vi "Initialize Transfers.vi"(7 "enable buffer conversion":bool, 8 "error in (no error)":errorcluster, 11 "transfer configurations":T1[](array[typedef]) {"channels"."string offset" format="%d bytes"}) -> (0 "error out":errorcluster, 3 "transfers":T6[](array[typedef]))   [LabVIEW 2017, in "DSF Core.lvlib" / "DSF PXImc Transceiver.lvclass"]
uses:
  DSF PXImc Transceiver.lvclass
  PXImc Transfer Data.ctl
  Typedefs/DSF Engine Transfer Configuration.ctl
  Typedefs/DSF Byte Order.ctl
  Typedefs/DSF Settings Info.ctl
  Typedefs/DSF Engine Channel Configuration.ctl
  Typedefs/DSF Data Type.ctl
  Classes/Configuration/Required Buffer Size (Transfer).vi
  Bad Setting Error.vi
  Classes/Configuration/Configuration Session.lvclass
  DSF Core.lvlib
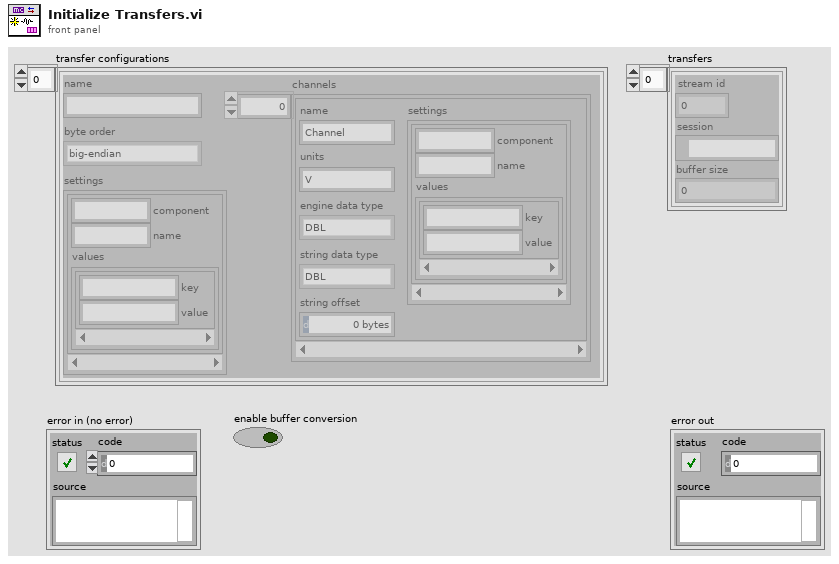
[diagram p1: front panel]
types:
  T1 = typedef "DSF Core.lvlib/DSF Engine Transfer Configuration.ctl" = cluster{"name":string, "byte order":T2, "settings":T3, "channels":T4[]}
  T2 = typedef "DSF Core.lvlib/DSF Byte Order.ctl" = enum8{"big-endian", "little-endian"}
  T3 = typedef "DSF Core.lvlib/DSF Settings Info.ctl" = cluster{"component":string, "name":string, "values":cluster{"key":string, "value":string}[]}[]
  T4 = typedef "DSF Core.lvlib/DSF Engine Channel Configuration.ctl" = cluster{"string offset":u64, "name":string, "units":string, "engine data type":T5, "string data type":T5, "settings":T3}
  T5 = typedef "DSF Core.lvlib/DSF Data Type.ctl" = enum8{"Bool", "SGL", "DBL", "I8", "I16", "I32", "I64", "U8", "U16", "U32", "U64"}
  T6 = typedef "DSF Core.lvlib/DSF PXImc Transceiver.lvclass/PXImc Transfer Data.ctl" = cluster{"stream id":u16, "session":refnum<k21>, "buffer size":u64}
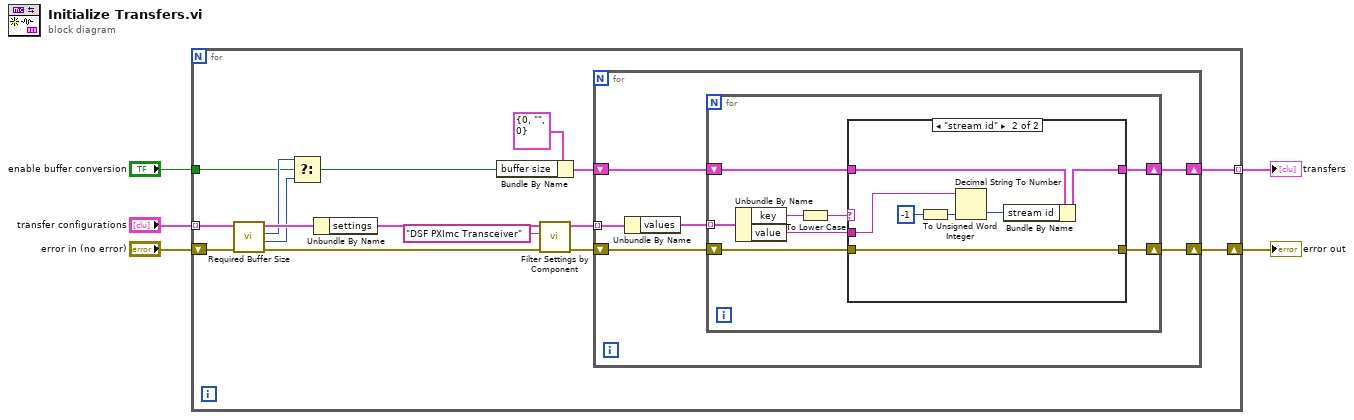
[diagram p0: block diagram]
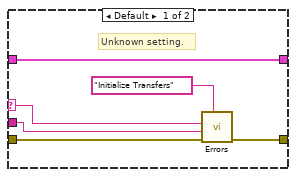
[diagram p2: hidden frame]
diagram:
  n1 = for {
    tunnel: "transfer configurations" -> [w13] mode=indexing
    tunnel: [w17] -> w3 mode=indexing
    shift-right: [w16] -> w4
    shift-left: "error in (no error)" -> [w12]
    tunnel: "enable buffer conversion" -> [w7]
    n2 = call-poly "Required Buffer Size.vi"("error in (no error)"=w12, "Transfer Configuration in"=w13) -> ("error out"=w10:errorcluster, "engine buffer size"=w8:u64, "string buffer size"=w9:u64, "Transfer Configuration out"=w11:T1)  [unwired: 6 in]
    n3 = Select(t=w9, s=w7, f=w8) -> (s? t:f=w6:u64)
    n4 = Unbundle By Name(w11) -> ("settings"=w21:T3)
    n5 = Bundle By Name(cluster=T6 {"stream id"=0, "session"="", "buffer size"=0} ("PXImc Transfer"), "buffer size"=w6) -> (w14:T6)
    n6 = call "Filter Settings by Component.vi"("error in (no error)"=w10, "component"="DSF PXImc Transceiver", "settings"=w21) -> ("error out"=w18:errorcluster, "filtered settings"=w19:T3)  [unwired: 7 in]
    n7 = for {
      tunnel: w19 -> [w27] mode=indexing
      shift-right: [w22] -> w16
      shift-left: w18 -> [w25]
      shift-right: [w23] -> w17
      shift-left: w14 -> [w24]
      n8 = Unbundle By Name(w27) -> ("values"=w26:cluster{"key":string, "value":string}[])
      n9 = for {
        tunnel: w26 -> [w35] mode=indexing
        shift-right: [w28] -> w22
        shift-left: w25 -> [w31]
        shift-right: [w29] -> w23
        shift-left: w24 -> [w30]
        n10 = Unbundle By Name(w35) -> ("key"=w34:string, "value"=w32:string)
        n11 = To Lower Case(string=w34) -> (all lower case string=w33:string)
        n12 = case shown="\"stream id\"" w33 {
          selector: w33 -> [w37 _]
          tunnel: w32 -> [w38 w48]
          tunnel: w31 -> [w40 w42]
          tunnel: w30 -> [w41 w44]
          tunnel: [w41 w43] -> w29
          tunnel: [w39 w42] -> w28
          frame Default {
            # "Unknown setting."
            n13 = call-poly "Errors.vi"("vi name"="Initialize Transfers", "error in (no error)"=w40, "value"=w38, "key"=w37) -> ("error out"=w39:errorcluster)  [unwired: 6 in, 1 out]
          }
          frame "stream id" {
            n14 = To Unsigned Word Integer(number=i16 -1 ("default (0 I32)")) -> (unsigned 16bit integer=w46:u16)
            n15 = Decimal String To Number(string=w48, default (0L)=w46) -> (number=w45:u16)  [unwired: 1 in, 1 out]
            n16 = Bundle By Name(cluster=w44, "stream id"=w45) -> (w43:T6)
          }
        }
      }
    }
  }
  "error out" <- w4
  "transfers" <- w3
